vi "Adding transaction tests.vi"() -> ()   [LabVIEW 2023]
uses:
  SQLite DB Operator/SQLite DB Operator.lvclass
  DB Records/Expenses Tracker Transaction/Expenses Tracker Transaction.lvclass
  H:/Desktop/LabVIEW/LabView Repo/Expenses-Tracker-DB-Operator/DB Records/Expenses Tracker Record/Expenses Tracker Record.lvclass
  DB Records/Expenses Tracker Record/Public/Ctrls/Transaction.ctl
  DB Records/Expenses Tracker Category/Expenses Tracker Category.lvclass
  DB Records/Expenses Tracker Record/Public/Ctrls/Category.ctl
  SQLite DB Operator/SQLite DB Operator.lvclass/SQLite DB Operator.ctl
  <vilib>/drjdpowell/SQLite Library/SQL Connection/Execute SQL (No results).vi
  <vilib>/drjdpowell/SQLite Library/SQL Connection/Execute SQL.vi
  <vilib>/drjdpowell/SQLite Library/SQL Connection/Execute SQL (Single DBL).vi
  <vilib>/drjdpowell/SQLite Library/SQL Connection/Connection.lvclass
  <vilib>/drjdpowell/SQLite Library/SQLite.lvlib
  DB Records/Expenses Tracker Record/Expenses Tracker Record.lvclass
panel:
  out "Result Set":string[][](table) caption="Result Set (from first statement with results)"
  out "time stamp":timestamp
  in  "SQL":string
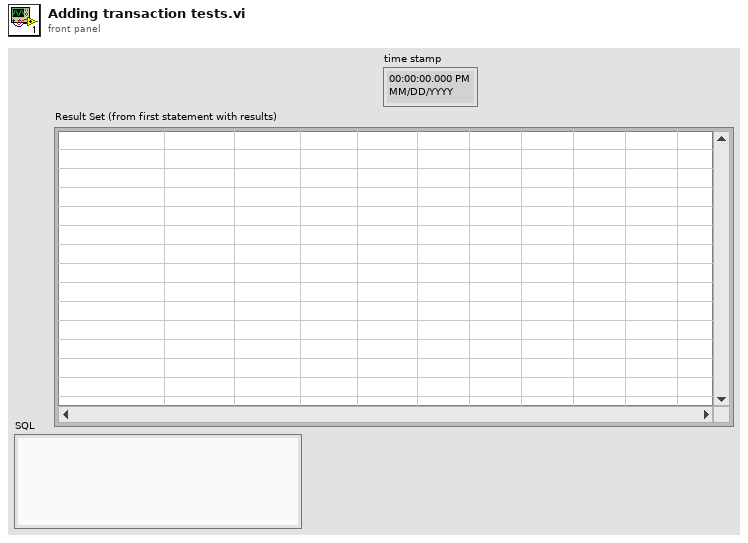
[diagram p1: front panel]
types:
  T1 = typedef "Expenses Tracker Record.lvclass/Category.ctl" = cluster{"ID":u32, "Name":string}
  T2 = typedef "Expenses Tracker Record.lvclass/Transaction.ctl" = cluster{"ID":u32, "Name":string, "Is_income":bool, "Value":dbl, "Amount":dbl, "Total":dbl, "Date_of_entry":timestamp, "Date":timestamp, "Last_update":timestamp, "Category":u32, "Subcategory":u32, "Cycle":u32, "Description":string}
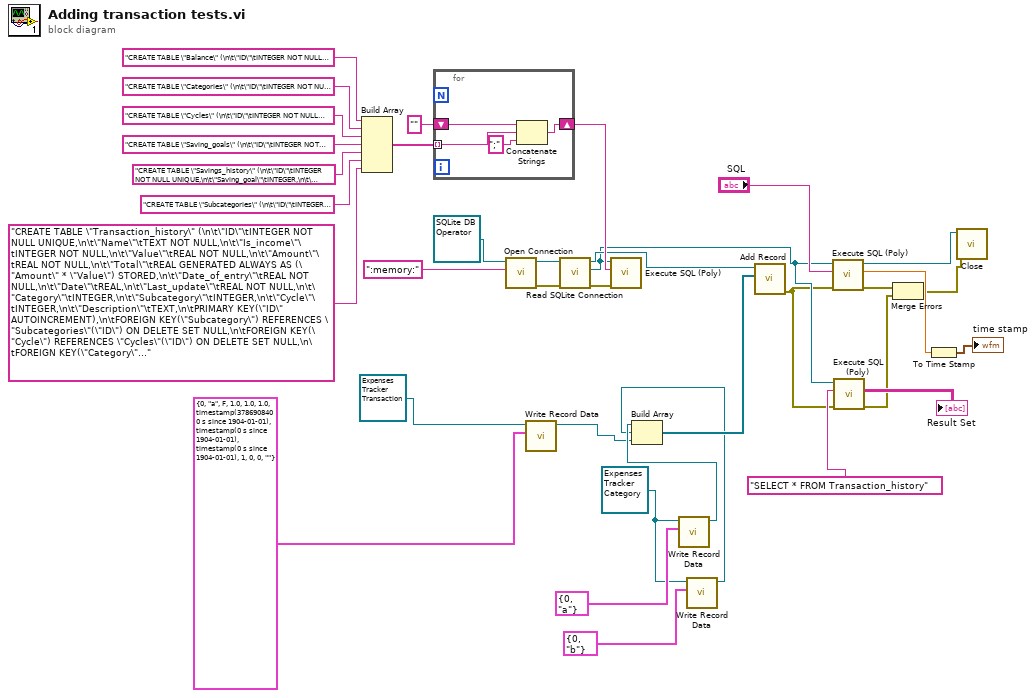
[diagram p0: block diagram]
diagram:
  w4 = refnum<class "Expenses Tracker Category.lvclass"> refnum ("Expenses Tracker Category")
  n1 = Build Array("CREATE TABLE \"Balance\" (\n\t\"ID\"\tINTEGER NOT NULL UNIQUE,\n\t\"Value\"\tREAL NOT NULL,\n\t\"Last_update\"\tREAL NOT NULL,\n\tPRIMARY KEY(\"ID\" AUTOINCREMENT)\n)", "CREATE TABLE \"Categories\" (\n\t\"ID\"\tINTEGER NOT NULL UNIQUE,\n\t\"Name\"\tTEXT NOT NULL UNIQUE,\n\tPRIMARY KEY(\"ID\" AUTOINCREMENT)\n)", "CREATE TABLE \"Cycles\" (\n\t\"ID\"\tINTEGER NOT NULL UNIQUE,\n\t\"Name\"\tTEXT NOT NULL UNIQUE,\n\t\"Day_of_occurence\"\tINTEGER NOT NULL,\n\t\"Description\"\tTEXT,\n\tPRIMARY KEY(\"ID\" AUTOINCREMENT)\n)", "CREATE TABLE \"Saving_goals\" (\n\t\"ID\"\tINTEGER NOT NULL UNIQUE,\n\t\"Is_active\"\tINTEGER NOT NULL,\n\t\"Name\"\tTEXT NOT NULL UNIQUE,\n\t\"Current_value\"\tREAL NOT NULL,\n\t\"Target_value\"\tREAL NOT NULL,\n\t\"Date_of_entry\"\tREAL NOT NULL,\n\t\"Due_date\"\tREAL,\n\t\"Last_update\"\tREAL NOT NULL,\n\t\"Description\"\tTEXT,\n\tPRIMARY KEY(\"ID\" AUTOINCREMENT)\n)", "CREATE TABLE \"Savings_history\" (\n\t\"ID\"\tINTEGER NOT NULL UNIQUE,\n\t\"Saving_goal\"\tINTEGER,\n\t\"Value\"\tREAL NOT NULL,\n\t\"Date_of_entry\"\tREAL NOT NULL,\n\t\"Description\"\tTEXT,\n\tFOREIGN KEY(\"Saving_goal\") REFERENCES \"Saving_goals\"(\"ID\") ON DELETE RESTRICT,\n\tPRIMARY KEY(\"ID\" AUTOINCREMENT)\n)", "CREATE TABLE \"Subcategories\" (\n\t\"ID\"\tINTEGER NOT NULL UNIQUE,\n\t\"Name\"\tTEXT NOT NULL,\n\t\"Category\"\tINTEGER NOT NULL,\n\tFOREIGN KEY(\"Category\") REFERENCES \"Categories\"(\"ID\") ON DELETE SET NULL,\n\tPRIMARY KEY(\"ID\" AUTOINCREMENT)\n)", "CREATE TABLE \"Transaction_history\" (\n\t\"ID\"\tINTEGER NOT NULL UNIQUE,\n\t\"Name\"\tTEXT NOT NULL,\n\t\"Is_income\"\tINTEGER NOT NULL,\n\t\"Value\"\tREAL NOT NULL,\n\t\"Amount\"\tREAL NOT NULL,\n\t\"Total\"\tREAL GENERATED ALWAYS AS (\"Amount\" * \"Value\") STORED,\n\t\"Date_of_entry\"\tREAL NOT NULL,\n\t\"Date\"\tREAL,\n\t\"Last_update\"\tREAL NOT NULL,\n\t\"Category\"\tINTEGER,\n\t\"Subcategory\"\tINTEGER,\n\t\"Cycle\"\tINTEGER,\n\t\"Description\"\tTEXT,\n\tPRIMARY KEY(\"ID\" AUTOINCREMENT),\n\tFOREIGN KEY(\"Subcategory\") REFERENCES \"Subcategories\"(\"ID\") ON DELETE SET NULL,\n\tFOREIGN KEY(\"Cycle\") REFERENCES \"Cycles\"(\"ID\") ON DELETE SET NULL,\n\tFOREIGN KEY(\"Category\") REFERENCES \"Categories\"(\"ID\") ON DELETE SET NULL\n)") -> (w25:string[])
  n2 = for {
    tunnel: w25 -> [w40] mode=indexing
    shift-right: [w38] -> w23
    shift-left: "" -> [w37]
    n3 = Concatenate Strings(w37, w40, ";" ("string")) -> (w38:string)
  }
  n4 = call-dynamic "Open Connection.vi"("DB Connection String/Path"=":memory:" ("db file"), "SQLite DB Operator In"=refnum<class "SQLite DB Operator.lvclass"> refnum ("SQLite DB Operator.lvclass")) -> ("Error Out"=w34:errorcluster, "SQLite DB Operator Out"=w35:refnum<class "SQLite DB Operator.lvclass">)  [unwired: 8 in]
  n5 = call-dynamic "Write Record Data.vi"("Record"=T2 {"ID"=0, "Name"="a", "Is_income"=FALSE, "Value"=1.0, "Amount"=1.0, "Total"=1.0, "Date_of_entry"=timestamp(3786908400 s since 1904-01-01), "Date"=timestamp(0 s since 1904-01-01), "Last_update"=timestamp(0 s since 1904-01-01), "Category"=1, "Subcategory"=0, "Cycle"=0, "Description"=""} ("Transaction"), "Expenses Tracker Transaction In"=refnum<class "Expenses Tracker Transaction.lvclass"> refnum ("Expenses Tracker Category")) -> ("Expenses Tracker Transaction Out"=w3:refnum<class "Expenses Tracker Transaction.lvclass">)  [unwired: 8 in, 1 out]
  n6 = call "Read SQLite Connection.vi"("Error In (no error)"=w34, "SQLite DB Operator In"=w35) -> ("Error Out"=w22:errorcluster, "SQLite.lvlib:Connection"=w13:refnum<class "Connection.lvclass">, "SQLite DB Operator out"=w21:refnum<class "SQLite DB Operator.lvclass">)  [unwired: 7 in]
  n7 = call-poly <vilib>:"Execute SQL (Poly).vi"("error in (no error)"=w22, "SQL"=w23, "SQLite Connection in"=w13) -> ()  [unwired: 7 in, 2 out]
  n8 = call-dynamic "Write Record Data.vi"("Record"=T1 {"ID"=0, "Name"="a"} ("Category"), "Expenses Tracker Category In"=w4) -> ("Expenses Tracker Category Out"=w17:refnum<class "Expenses Tracker Category.lvclass">)  [unwired: 8 in, 1 out]
  n9 = call-dynamic "Write Record Data.vi"("Record"=T1 {"ID"=0, "Name"="b"} ("Category"), "Expenses Tracker Category In"=w4) -> ("Expenses Tracker Category Out"=w2:refnum<class "Expenses Tracker Category.lvclass">)  [unwired: 8 in, 1 out]
  n10 = Build Array(w17, w2, w3) -> (w18:refnum<class "Expenses Tracker Record.lvclass">[])
  n11 = call-dynamic "Add Record.vi"("Expenses Tracker Records In"=w18, "SQLite DB Operator In"=w21) -> ("Error Out"=w10:errorcluster)  [unwired: 7 in, 2 out]
  n12 = call-poly <vilib>:"Execute SQL (Poly).vi"("error in (no error)"=w10, "SQL"="SQL", "SQLite Connection in"=w13) -> ("error out"=w8:errorcluster, "Result"=w15:dbl, "SQLite Connection"=w9:refnum<class "Connection.lvclass">)  [unwired: 6 in]
  n13 = call-poly <vilib>:"Execute SQL (Poly).vi"("error in (no error)"=w10, "SQL"="SELECT * FROM Transaction_history", "SQLite Connection in"=w13) -> ("error out"=w6:errorcluster, "Result Set"=→"Result Set":string[][])  [unwired: 5 in, 2 out]
  n14 = Merge Errors(w8, w6) -> (w7:errorcluster)
  n15 = To Time Stamp(1:w15) -> (0:→"time stamp":timestamp)
  n16 = call-dynamic "Close.vi"("error in (no error)"=w7, "SQLite Connection in"=w9) -> ()  [unwired: 9 in, 1 out]
